vi "Goal Vision Calculations V4.vi"(10 "Target Height (in)":dbl=11.0) -> (1 "Angle":dbl=0.20104217529296875, 2 "distance ft":dbl=3.9967712350677553)   [LabVIEW 2017]
uses:
  <vilib>/Rock Robotics/Network Tables/NT Read Number.vi
  <vilib>/Rock Robotics/Network Tables/NT Write Number.vi
panel:
  in  "Y axis field of view (deg)":dbl=34.3
  in  "Camera Angle (deg)":dbl=48.0
  in  "Camera Height (in)":dbl=50.0
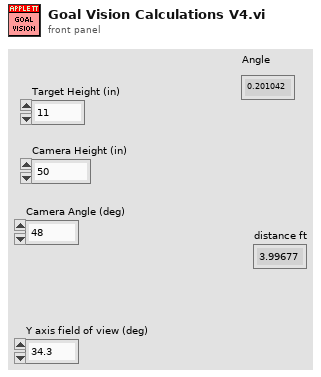
[diagram p1: front panel]
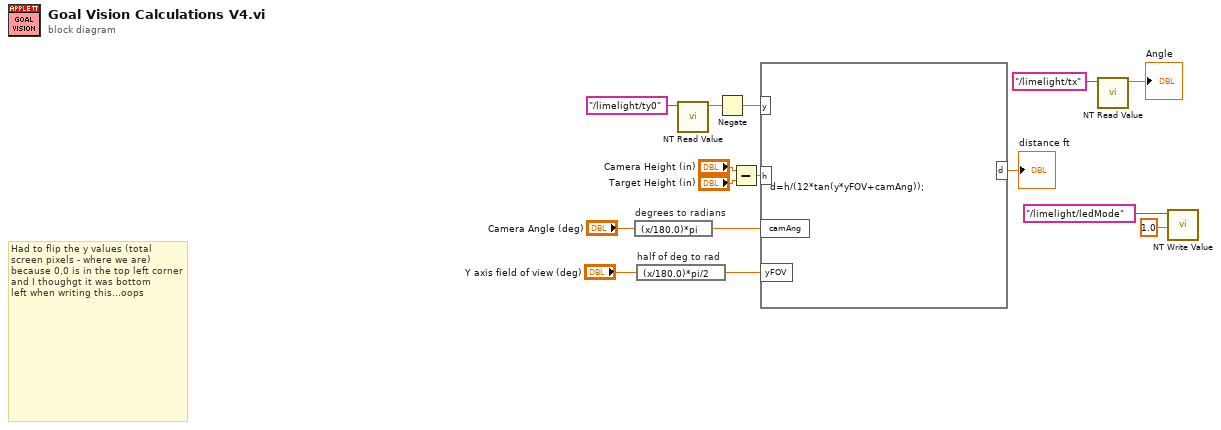
[diagram p0: block diagram]
diagram:
  # "Had to flip the y values (total screen pixels - where we are) because 0,0 is in the top left corner and I thoughgt it was bottom \nleft when writing this...oops"
  n1 = expression code="(x/180.0)*pi" "degrees to radians"("Camera Angle (deg)") -> (w12:dbl)
  n2 = expression code="(x/180.0)*pi/2" "half of deg to rad"("Y axis field of view (deg)") -> (w13:dbl)
  n3 = call-poly <vilib>:"NT Read Value.vi"("Name"="/limelight/ty0") -> ("Numeric"=w7:dbl)  [unwired: 9 in, 1 out]
  n4 = Negate(x=w7) -> (-x=w6:dbl)
  n5 = Subtract(x="Camera Height (in)", y="Target Height (in)") -> (x-y=w11:dbl)
  n6 = formula code="d=h/(12*tan(y*yFOV+camAng));"("y"=w6, "h"=w11, "camAng"=w12, "yFOV"=w13) -> ("d"=→"distance ft":dbl)
  n7 = call-poly <vilib>:"NT Read Value.vi"("Name"="/limelight/tx") -> ("Numeric"=→"Angle":dbl)  [unwired: 9 in, 1 out]
  n8 = call-poly <vilib>:"NT Write Value.vi"("Numeric"=1.0, "Name"="/limelight/ledMode") -> ()  [unwired: 9 in, 1 out]
